vi "Diagnostics.TCP.Connect.Engine.vi"(8 "error in (no error)":errorcluster, 11 "State Variables":T1={"TCP Refs"={"Connection List"=refnum, "listener ID"=refnum}, "Parameters"={"Properties"={"Name"="", "CAN"={"CAN Interface"=enum."CAN0", "Baud Rate"=0, "Diagnostic Protocol"=enum."GMLAN", "Transport Protocol"=enum."ISO TP - Normal Mode", "Transmit ID"=0, "Receive ID"=0, "Transmit Extension"=0, "Receive Extension"=0, "Receive UUDT ID"=0, "Enable Stream"=TRUE, "VW TP Channel ID"=0, "Security"={"Source DLL Path"=path "", "Security Level"=1, "Target DLL Path"=path ""}, "Fill Frame"=FALSE, "Fill Byte"=255, "Termination"=FALSE}, "986x"={"Enable"=FALSE, "RIO Device"=0, "Bitfile"=path ""}, "Reads"=[], "Frames Lookup"=variant, "Writes"=[], "DPIDs"=[], "DPID Lookup"=variant, "DTC descriptor"={"DTC Byte Length"=2, "Status Byte Length"=1, "Add Data Byte Length"=1, "Byte Order"=enum."Motorola"}, "Created DTCs"=0}, "ChanRefs"={"ToVS.Reads"={"Name"="", "Write to VS Engine FIFO"=refnum, "Pairs"={"Refs"=[], "Values"=[]}}, "ToVS.DTCs"={"Name"="", "Write to VS Engine FIFO"=refnum, "Pairs"={"Refs"=[], "Values"=[]}}, "ToVS.DTCCount"={"Name"="", "Write to VS Engine FIFO"=refnum, "Pairs"={"Refs"=[], "Values"=[]}}, "ToVS.Status"={"Name"="", "Write to VS Engine FIFO"=refnum, "Pairs"={"Refs"=[], "Values"=[]}}, "FromVS.Writes"={"Name"="", "Read from VS Engine FIFO"=refnum, "Pairs"={"Refs"=[], "Values"=[]}}, "Cmds"={"Name"="", "Write to VS Engine FIFO"=refnum, "Read from VS Engine FIFO"=refnum, "Pairs"={"Chan Refs"=[], "Prev. Values"=[]}}, "Triggers"={"Name"="", "Write to VS Engine FIFO"=refnum, "Read from VS Engine FIFO"=refnum, "Pairs"={"Chan Refs"=[], "Prev. Values"=[]}}}}, "ADCS Connection"={"Diag CAN Handle"=0, "Transport Protocol"=enum."ISO TP - Normal Mode", "Receive Address Extension"=0, "Transmit Address Extension"=0, "Receive CAN Id"=0, "Transmit CAN Id"=0, "Diag CAN Queue"=refnum, "Log Frames ?"=FALSE, "My TP Address"=0, "Other TP Address"=0, "T1"=0, "T2"=0, "T3"=0, "T4"=0, "Tx SN"=0, "Block Size"=0, "Rx SN"=0, "VW TP Initialized?"=FALSE, "Tx block no"=0, "baud rate"=0, "Interface"="", "Channel Diag CAN Handle"=0, "UDP Connection ID"=refnum, "TCP Connection ID"=refnum, "Target IP Addr"=0, "Source Address"=0, "Target Address"=0, "Send Header NACK?"=FALSE, "DLL Handle"=0, "NAD"=0, "Time Stamp read first"=0.0, "Time Stamp read last"=0.0, "Time Stamp write first"=0.0, "Time Stamp write last"=0.0, "Time Stamp write"=0.0, "Time Stamp read"=0.0}, "XNET References"={"Database"="", "GMLAN DPID Session"="", "Cluster"=""}, "BufferedCmds"=refnum, "XNETEngine (GMLAN)"=refnum, "Process"=refnum} {"Parameters"."ChanRefs"."Triggers"."Pairs"."Chan Refs" format="%.0x"; "Parameters"."ChanRefs"."Cmds"."Pairs"."Chan Refs" format="%.0x"; "Parameters"."ChanRefs"."ToVS.Status"."Pairs"."Refs" format="%.0x"; "Parameters"."ChanRefs"."ToVS.DTCCount"."Pairs"."Refs" format="%.0x"; "Parameters"."ChanRefs"."ToVS.DTCs"."Pairs"."Refs" format="%.0x"; "Parameters"."ChanRefs"."ToVS.Reads"."Pairs"."Refs" format="%.0x"; "Parameters"."Properties"."Writes"."Signals"."Byte Order" items=["Little Endian", "Big Endian"]; "Parameters"."Properties"."Writes"."Signals"."Data Type" items=["Signed", "Unsigned", "IEEE Float"]; "Parameters"."Properties"."CAN"."Fill Byte" format="%.0x"; "Parameters"."Properties"."CAN"."VW TP Channel ID" format="%.0x"; "Parameters"."Properties"."CAN"."Receive UUDT ID" format="%.0x"; "Parameters"."Properties"."CAN"."Receive Extension" format="%.0x"; "Parameters"."Properties"."CAN"."Transmit Extension" format="%.0x"; "Parameters"."Properties"."CAN"."Receive ID" format="%.0x"; "Parameters"."Properties"."CAN"."Transmit ID" format="%.0x"; "Parameters"."Properties"."Reads"."Signals"."Byte Order" items=["Little Endian", "Big Endian"]; "Parameters"."Properties"."Reads"."Signals"."Data Type" items=["Signed", "Unsigned", "IEEE Float"]}) -> (0 "error out":errorcluster)   [LabVIEW 2015, in "Diagnostics Addon Engine.lvlib"]
uses:
  Diagnostics Addon Engine.lvlib
  Types/Diagnostics.State.ctl
  <vilib>/NI/NI VeriStand Inline Async API/_VS Inline Async API/Process/Process.lvclass
  Types/TCP.Refs.ctl
  STM/STM Lookup Table Ref.ctl
  Types/Engine.State.ctl
  Shared/Types/SysDef.Compile.Properties.ctl
  Shared/Types/CAN.ctl
  Shared/Types/CAN.Interface.ctl
  Shared/Types/Protocol.ctl
  Shared/Types/Transport.ctl
  Shared/Types/Security.ctl
  Shared/Types/986x.ctl
  Shared/Types/Frame.Compile.ctl
  Shared/Types/Type.ctl
  Shared/Types/Signal.ctl
  Shared/Types/DPID.ctl
  Shared/Types/DPID.Rate.ctl
  Shared/Types/DTCDescriptor.ctl
  Types/Engine.Refs.ctl
  Inline Async API/Controls/Write To VS Engine.ctl
  <vilib>/NI Veristand/Custom Device API/Data Reference.ctl
  Inline Async API/Controls/Read From VS Engine.ctl
  <vilib>/NI Veristand/Custom Device API/Block Data Reference.ctl
  Inline Async API/Controls/ReadWrite Data.ctl
  <vilib>/Automotive Diagnostic Command Set/Diagnostic Transport.llb/Diag Reference.ctl
  <vilib>/Automotive Diagnostic Command Set/Diagnostic Transport.llb/Transport Protocol Selector.ctl
  <vilib>/Automotive Diagnostic Command Set/Diagnostic Transport.llb/Diag CAN Frame Log.ctl
  Types/XNET.Refs.ctl
  <vilib>/NI/AMC/Message Queue.ctl
  <vilib>/NI/AMC/Message.ctl
  <vilib>/NI/Tools/Keyed Array/KeyedArray.ctl
  STM/TCP/stm_TCP Read Options.ctl
  STM/Connection Manager/stm_TCPConnectionMethod.ctl
  STM/Connection Manager/stm_TCPConnectionProperties.ctl
  <vilib>/NI/NI VeriStand Inline Async API/_VS Inline Async API/Process/Process.lvclass/Process.ctl
  <vilib>/NI/NI VeriStand Inline Async API/_VS Inline Async API/Error Handling Process/SubVIs/Error.ConvertArray.vi
  STM/TCP/STM Read Meta Data (TCP Ref).vi
  <vilib>/NI Veristand/Custom Device Tools/Custom Device Utility Library/Custom Device Utility Library.lvlib
  Shared/Diagnostics Addon Shared.lvlib
  <vilib>/NI VeriStand/Custom Device API/Custom Device API.lvlib
  <vilib>/NI/Tools/Keyed Array/Tools_KeyedArray.lvlib
  <vilib>/NI/AMC/AMC.lvlib
  <vilib>/addons/Automotive Diagnostic Command Set/NI_Automotive Diagnostic Command Set.lvlib
  Inline Async API/Inline Async API.lvlib
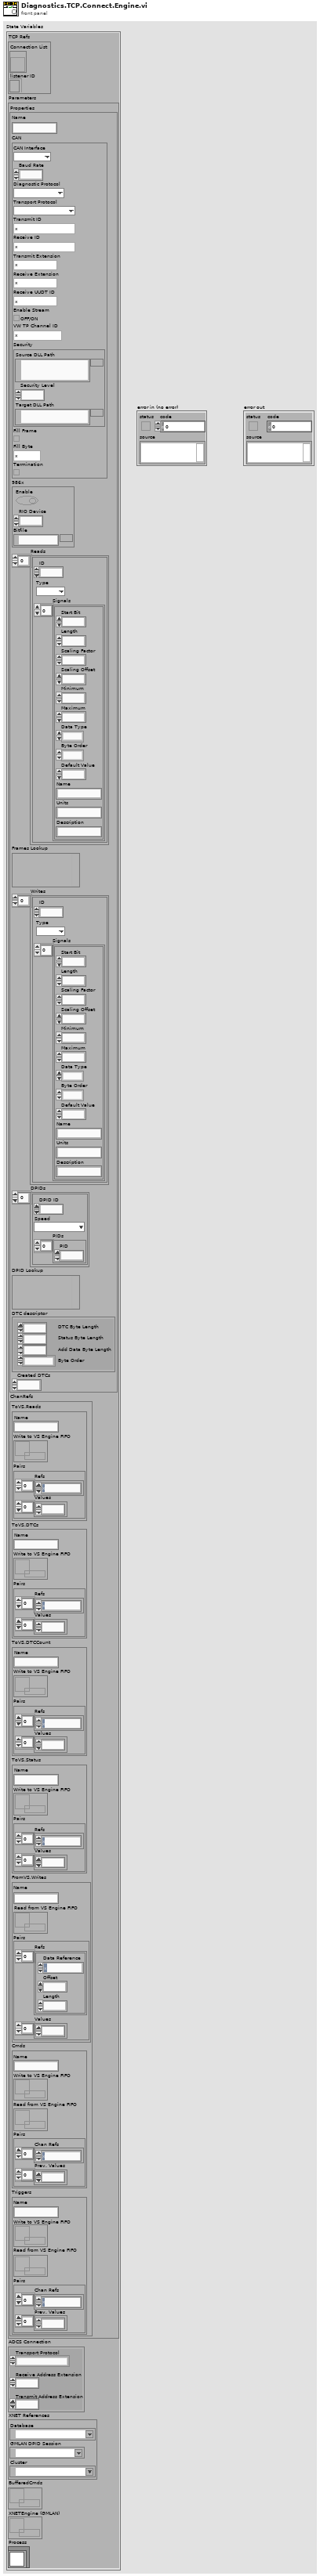
[diagram p1: front panel]
types:
  T1 = typedef "Diagnostics Addon Engine.lvlib/Diagnostics.State.ctl" = cluster{"TCP Refs":T2, "Parameters":T4, "ADCS Connection":T24, "XNET References":T26, "BufferedCmds":T27, "XNETEngine (GMLAN)":T27, "Process":refnum<class "Process.lvclass">}
  T2 = typedef "Diagnostics Addon Engine.lvlib/TCP.Refs.ctl" = cluster{"Connection List":T3, "listener ID":refnum<k5>}
  T3 = typedef "Diagnostics Addon Engine.lvlib/STM Lookup Table Ref.ctl" = refnum<vi>
  T4 = typedef "Diagnostics Addon Engine.lvlib/Engine.State.ctl" = cluster{"Properties":T5, "ChanRefs":T18}
  T5 = typedef "Diagnostics Addon Shared.lvlib/SysDef.Compile.Properties.ctl" = cluster{"Name":string, "CAN":T6, "986x":T11, "Reads":T12[], "Frames Lookup":variant, "Writes":T12[], "DPIDs":T15[], "DPID Lookup":variant, "DTC descriptor":T17, "Created DTCs":u32}
  T6 = typedef "Diagnostics Addon Shared.lvlib/CAN.ctl" = cluster{"CAN Interface":T7, "Baud Rate":u32, "Diagnostic Protocol":T8, "Transport Protocol":T9, "Transmit ID":u32, "Receive ID":u32, "Transmit Extension":u8, "Receive Extension":u8, "Receive UUDT ID":u32, "Enable Stream":bool, "VW TP Channel ID":u32, "Security":T10, "Fill Frame":bool, "Fill Byte":u8, "Termination":bool}
  T7 = typedef "Diagnostics Addon Shared.lvlib/CAN.Interface.ctl" = enum16{"CAN0", "CAN1", "CAN2", "CAN3", "CAN4", "CAN5", "CAN6", "CAN7", "CAN8", "CAN9", "CAN10", "CAN11", "CAN12", "CAN13", "CAN14", "CAN15", "CAN16", "CAN17", "CAN18", "CAN19", "CAN20", "CAN21", "CAN22", "CAN23", "CAN24", "CAN25", "CAN26", "CAN27", "CAN28", "CAN29", "CAN30", "CAN31", "CAN32", "CAN33", "CAN34", "CAN35", "CAN36", "CAN37", "CAN38", "CAN39", "CAN40", "CAN41", "CAN42", "CAN43", "CAN44", "CAN45", "CAN46", "CAN47", "CAN48", "CAN49", "CAN50", "CAN51", "CAN52", "CAN53", "CAN54", "CAN55", "CAN56", "CAN57", "CAN58", "CAN59", "CAN60", "CAN61", "CAN62", "CAN63", "CAN 256 (Virtual)", "CAN 257 (Virtual)"}
  T8 = typedef "Diagnostics Addon Shared.lvlib/Protocol.ctl" = enum16{"GMLAN", "KWP-2000", "UDS", "User-Defined"}
  T9 = typedef "Diagnostics Addon Shared.lvlib/Transport.ctl" = enum16{"ISO TP - Normal Mode", "ISO TP - Mixed Mode", "VW TP 2.0", "Diagnostics on IP"}
  T10 = typedef "Diagnostics Addon Shared.lvlib/Security.ctl" = cluster{"Source DLL Path":path, "Security Level":u8, "Target DLL Path":path}
  T11 = typedef "Diagnostics Addon Shared.lvlib/986x.ctl" = cluster{"Enable":bool, "RIO Device":u16, "Bitfile":path}
  T12 = typedef "Diagnostics Addon Shared.lvlib/Frame.Compile.ctl" = cluster{"ID":u32, "Type":T13, "Signals":T14[]}
  T13 = typedef "Diagnostics Addon Shared.lvlib/Type.ctl" = enum16{"DID", "CDID", "PID", "CPID", "Read Memory", "Write Memory", "DTC Control", "IO Cmd", "IO Resp", "Routine Start Cmd", "Routine Start Resp", "Routine Request Cmd", "Routine Request Resp", "Routine Stop Cmd", "Routine Stop Resp", "UserDefined Cmd", "UserDefined Rsp"}
  T14 = typedef "Diagnostics Addon Shared.lvlib/Signal.ctl" = cluster{"Start Bit":u32, "Length":u32, "Scaling Factor":dbl, "Scaling Offset":dbl, "Minimum":dbl, "Maximum":dbl, "Data Type":u32, "Byte Order":u32, "Default Value":dbl, "Name":string, "Units":string, "Description":string}
  T15 = typedef "Diagnostics Addon Shared.lvlib/DPID.ctl" = cluster{"DPID ID":u8, "Speed":T16, "PIDs":u16[]}
  T16 = typedef "Diagnostics Addon Shared.lvlib/DPID.Rate.ctl" = enum16{"Slow", "Medium", "Fast"}
  T17 = typedef "Diagnostics Addon Shared.lvlib/DTCDescriptor.ctl" = cluster{"DTC Byte Length":i32, "Status Byte Length":i32, "Add Data Byte Length":i32, "Byte Order":enum16{"Motorola", "Intel"}}
  T18 = typedef "Diagnostics Addon Engine.lvlib/Engine.Refs.ctl" = cluster{"ToVS.Reads":T19, "ToVS.DTCs":T19, "ToVS.DTCCount":T19, "ToVS.Status":T19, "FromVS.Writes":T21, "Cmds":T23, "Triggers":T23}
  T19 = typedef "Diagnostics Addon Engine.lvlib/Inline Async API.lvlib/Write To VS Engine.ctl" = cluster{"Name":string, "Write to VS Engine FIFO":refnum<k33>, "Pairs":cluster{"Refs":T20[], "Values":dbl[]}}
  T20 = typedef "Custom Device API.lvlib/Data Reference.ctl" = i32
  T21 = typedef "Diagnostics Addon Engine.lvlib/Inline Async API.lvlib/Read From VS Engine.ctl" = cluster{"Name":string, "Read from VS Engine FIFO":refnum<k33>, "Pairs":cluster{"Refs":T22[], "Values":dbl[]}}
  T22 = typedef "Custom Device API.lvlib/Block Data Reference.ctl" = cluster{"Data Reference":T20, "Offset":u64, "Length":u64}
  T23 = typedef "Diagnostics Addon Engine.lvlib/Inline Async API.lvlib/ReadWrite Data.ctl" = cluster{"Name":string, "Write to VS Engine FIFO":refnum<k33>, "Read from VS Engine FIFO":refnum<k33>, "Pairs":cluster{"Chan Refs":T20[], "Prev. Values":dbl[]}}
  T24 = typedef "NI_Automotive Diagnostic Command Set.lvlib/Diag Reference.ctl" = cluster{"Diag CAN Handle":u32, "Transport Protocol":T25, "Receive Address Extension":u8, "Transmit Address Extension":u8, "Receive CAN Id":u32, "Transmit CAN Id":u32, "Diag CAN Queue":refnum<queue>, "Log Frames ?":bool, "My TP Address":u8, "Other TP Address":u8, "T1":u16, "T2":u16, "T3":u16, "T4":u16, "Tx SN":u8, "Block Size":u8, "Rx SN":u8, "VW TP Initialized?":bool, "Tx block no":u8, "baud rate":u32, "Interface":string, "Channel Diag CAN Handle":u32, "UDP Connection ID":refnum<k16>, "TCP Connection ID":refnum<k5>, "Target IP Addr":u32, "Source Address":u16, "Target Address":u16, "Send Header NACK?":bool, "DLL Handle":u32, "NAD":u8, "Time Stamp read first":dbl, "Time Stamp read last":dbl, "Time Stamp write first":dbl, "Time Stamp write last":dbl, "Time Stamp write":dbl, "Time Stamp read":dbl}
  T25 = typedef "NI_Automotive Diagnostic Command Set.lvlib/Transport Protocol Selector.ctl" = enum16{"ISO TP - Normal Mode", "ISO TP - Mixed Mode", "VW TP 2.0", "Diagnostics on IP", "ISO TP LIN"}
  T26 = typedef "Diagnostics Addon Engine.lvlib/XNET.Refs.ctl" = cluster{"Database":refnum<k21>, "GMLAN DPID Session":refnum<k21>, "Cluster":refnum<k21>}
  T27 = typedef "AMC.lvlib/Message Queue.ctl" = refnum<queue>
  T28 = typedef "Diagnostics Addon Engine.lvlib/stm_TCP Read Options.ctl" = cluster{"Ignore Timeout Error":bool, "timeout ms (1000)":i32}
  T29 = typedef "Diagnostics Addon Engine.lvlib/stm_TCPConnectionProperties.ctl" = cluster{"Name":string, "Address":string, "Custom":string}
  T30 = typedef "Diagnostics Addon Engine.lvlib/stm_TCPConnectionMethod.ctl" = enum16{"Initialize", "Add Connection", "Set Properties", "Get Connection(s)", "Remove Connection", "Remove All Connections", "Get Connection Count"}
  T31 = typedef "Diagnostics Addon Engine.lvlib/stm_TCP Connection Info.ctl" = cluster{"connection ID":refnum<k5>, "Meta data":T32[]}
  T32 = typedef "Diagnostics Addon Engine.lvlib/stm_MetaDataElement.ctl" = string
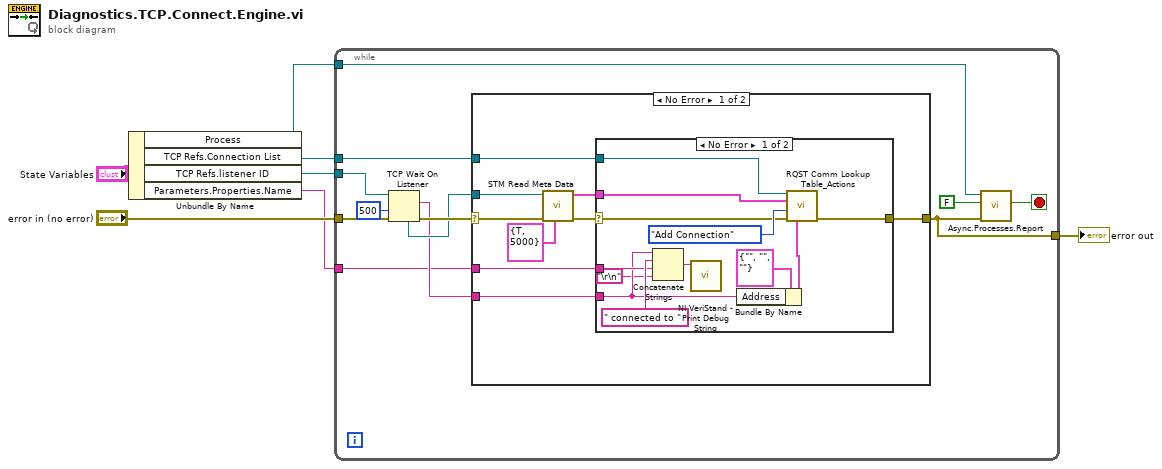
[diagram p0: block diagram]
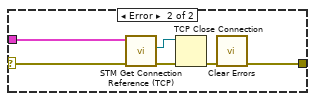
[diagram p2: hidden frame]
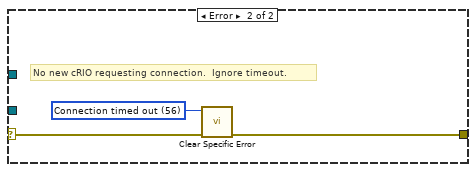
[diagram p3: hidden frame]
diagram:
  n1 = Unbundle By Name("State Variables") -> ("Process"=w7:refnum<class "Process.lvclass">, "TCP Refs.Connection List"=w5:T3, "TCP Refs.listener ID"=w6:refnum<k5>, "Parameters.Properties.Name"=w1:string)
  n2 = while {
    tunnel: "error in (no error)" -> [w19]
    tunnel: w6 -> [w18]
    tunnel: w7 -> [w11]
    tunnel: [w9] -> w2
    tunnel: w5 -> [w13]
    tunnel: w1 -> [w12]
    stop <- w10 stop-if-true
    n3 = TCP Wait On Listener(8:w19, 9:500 ("timeout ms (wait forever: -1)"), 11:w18) -> (0:w16:errorcluster, 2:w14:string, 4:w15:refnum<k5>)  [unwired: 1 in, 2 out]
    n4 = case shown="No Error" w16 {
      selector: w16 -> [w28 w49]
      tunnel: w15 -> [w22 _]
      tunnel: [w26 w48] -> w9
      tunnel: w14 -> [w24 _]
      tunnel: w13 -> [w25 _]
      tunnel: w12 -> [w23 _]
      frame No Error {
        n5 = call-poly "STM Read Meta Data.vi"("Options"=T28 {"Ignore Timeout Error"=TRUE, "timeout ms (1000)"=5000}, "error in"=w28, "connection ID"=w22) -> ("error out"=w21:errorcluster, "Connection Info Out"=w20:T31)  [unwired: 6 in, 1 out]
        n6 = case shown="No Error" w21 {
          selector: w21 -> [w36 w45]
          tunnel: w25 -> [w34 _]
          tunnel: w20 -> [w35 w44]
          tunnel: [w37 w46] -> w26
          tunnel: w24 -> [w30 _]
          tunnel: w23 -> [w31 _]
          frame No Error {
            n7 = Concatenate Strings(w30, " connected to " ("string"), w31, "\r\n") -> (w32:string)
            n8 = call <vilib>:"NI VeriStand - Print Debug String.vi"("Message"=w32) -> ()  [unwired: 10 in, 1 out]
            n9 = Bundle By Name(cluster=T29 {"Name"="", "Address"="", "Custom"=""} ("Properties In"), "Address"=w30) -> (w40:T29)
            n10 = call "RQST Comm Lookup Table_Actions.vi"("ref in"=w34, "Connection In"=w35, "Method"=stm_TCPConnectionMethod."Add Connection", "error in (no error)"=w36, "Properties In"=w40) -> ("error out"=w37:errorcluster)  [unwired: 4 in, 6 out]
          }
          frame Error {
            n11 = call "STM Get Connection Reference (TCP).vi"("error in"=w45, "Connection Info"=w44) -> ("error out"=w43:errorcluster, "connection ID out"=w42:refnum<k5>)  [unwired: 7 in, 1 out]
            n12 = TCP Close Connection(connection ID=w42, error in (no error)=w43) -> (error out=w41:errorcluster)  [unwired: 1 in, 1 out]
            n13 = call <vilib>:"Clear Errors.vi"("error in (no error)"=w41) -> ("error out"=w46:errorcluster)  [unwired: 5 in, 1 out]
          }
        }
      }
      frame Error {
        w47 = 56 items=["No Error", "Argument Error", "Memory Full", "Out of Zone", "End of File", "File Already Open", "Generic File IO Error", "File Not Found", "File Permission Error", "Disk Full", "Duplicate Path", "Too Many Files Open", "Not Enabled", "Resource File Not Found", "Cannot Add Resource", "Resource Not Found", "Image Not Found", "Image Memory Error", "Pen Does Not Exist", "Config Bad Type", "Config Token Not Found", "Config Parse Error", "Config Memory Error", "Bad External Code Format", "Bad External Code Offset", "External Code Not Present", "Null Window", "Destroy Window Mixup", "Null Menu", "Print Aborted", "Bad Print Record", "Print Driver Error", "Windows Error During Print", "Memory Error During Print", "Print Dialog Error", "Generic Print Error", "Invalid Device Refnum", "Device Not Found", "Device Parameter Error", "Device Unit Error", "Can't Open Device", "Device Call Aborted", "Generic Error", "Cancelled By User", "Object ID Too Low", "Object ID Too High", "Object Not In Heap", "Unknown Heap", "Bad DefProc ID", "DefProc Not In Table", "Message Out Of Range", "Null Method", "Unknown Message", "Manager Call Not Supported", "Bad address", "Connection In progress", "Connection timed out", "Connection is already in progress", "Network attribute not supported", "Network error", "Address in use", "System out of memory", "Connection aborted", "Connection refused", "Connection is not connected", "Connection is already connected", "Connection closed", "Initialize error (interapplication manager)", "Bad occurrence", "Wait on unbound occurrence handler", "Occurrence queue overflow", "Bad path", "Semaphore not signaled", "Unrecognized type (interapplication manager)"] ("1st Error to Convert")
        # "No new cRIO requesting connection.  Ignore timeout."
        n14 = call "Clear Specific Error.vi"("error in (no error)"=w49, "code"=w47) -> ("error out"=w48:errorcluster)  [unwired: 9 out]
      }
    }
    n15 = call <vilib>:"Async.Processes.Report.vi"("Error"=w9, "Stop on Error?"=FALSE, "Process in"=w11) -> ("Stop"=w10:bool)  [unwired: 7 in, 1 out]
  }
  "error out" <- w2
